vi "Get Button Refnum.vi"(8 "error in (no error)":errorcluster, 11 "Button in":refnum<class "Button.lvclass">) -> (0 "error out":errorcluster, 2 "Bool Refnum":refnum<vi>, 3 "Button out":refnum<class "Button.lvclass">)   [LabVIEW 2020, in "Button.lvlib" / "Button.lvclass"]
uses:
  Button.lvclass
  Button.lvclass/Button.ctl
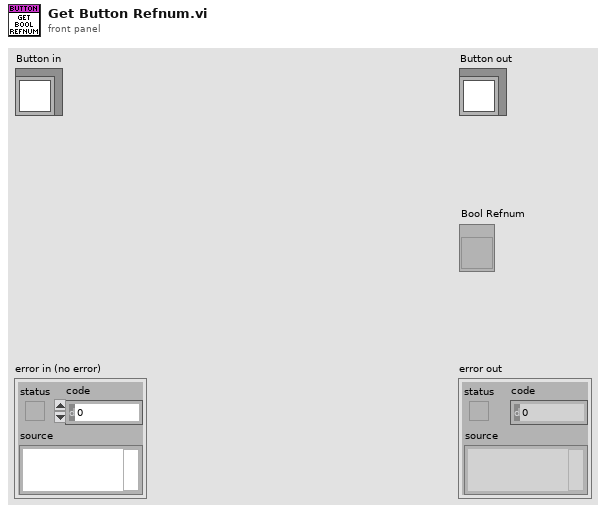
[diagram p1: front panel]
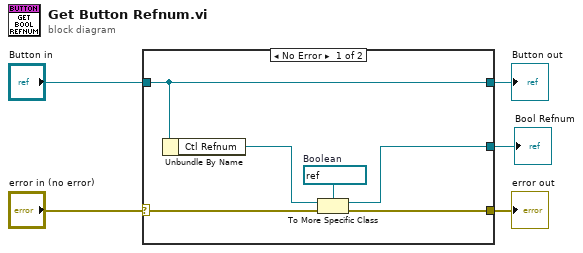
[diagram p0: block diagram]
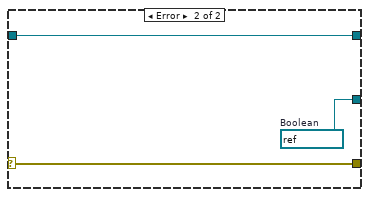
[diagram p2: hidden frame]
diagram:
  n1 = case shown="No Error" "error in (no error)" {
    selector: "error in (no error)" -> [w11 w14]
    tunnel: [w6 w14] -> w4
    tunnel: [w10 w13] -> w2
    tunnel: "Button in" -> [w10 w13]
    tunnel: [w7 w12] -> w1
    frame No Error {
      w8 = refnum<vi> refnum  # Boolean
      n2 = Unbundle By Name(w10) -> ("Ctl Refnum"=w9:refnum<vi>)
      n3 = To More Specific Class(target class=w8, reference=w9, error in=w11) -> (specific class reference=w7:refnum<vi>, error out=w6:errorcluster)
    }
    frame Error {
      w12 = refnum<vi> refnum  # Boolean
    }
  }
  "error out" <- w4
  "Button out" <- w2
  "Bool Refnum" <- w1
